vi "save_wav_as_txt.vi"(9 "文件夹名":string, 10 "txt名":string, 11 "wav":dbl[](array[numeric]) caption="一维数据") -> ()   [LabVIEW 2018]
uses:
  <vilib>/Utility/file.llb/Write Delimited Spreadsheet (DBL).vi
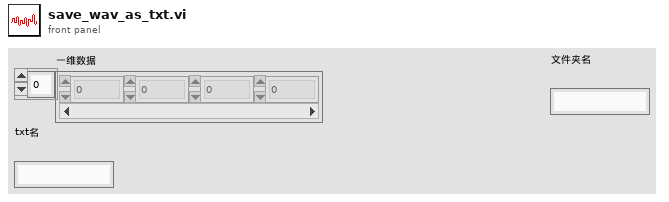
[diagram p1: front panel]
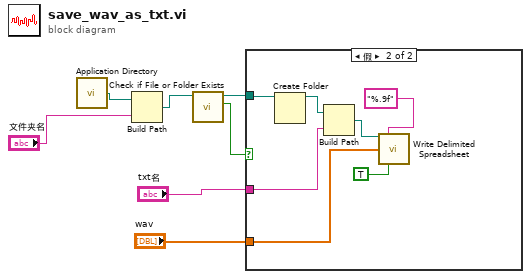
[diagram p0: block diagram]
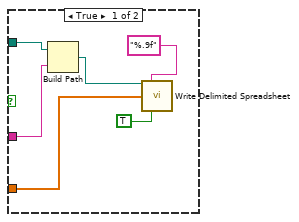
[diagram p2: hidden frame]
diagram:
  n1 = call <vilib>:"Application Directory.vi"() -> ("Application Directory"=w1:path)
  n2 = Build Path(base path=w1, name or relative path="文件夹名") -> (appended path=w6:path)
  n3 = call <vilib>:"Check if File or Folder Exists.vi"("path"=w6) -> ("file or folder exists?"=w5:bool, "dup path"=w3:path)  [unwired: 8 in, 1 out]
  n4 = case shown="假" w5 {
    tunnel: "wav" -> [w11 w18]
    tunnel: w3 -> [w10 w17]
    tunnel: "txt名" -> [w9 w15]
    frame True {
      n5 = Build Path(base path=w10, name or relative path=w9) -> (appended path=w8:path)
      n6 = call-poly <vilib>:"Write Delimited Spreadsheet.vi"("file path (dialog if empty)"=w8, "format (%.3f)"="%.9f", "1D data"=w11, "transpose? (no:F)"=TRUE) -> ()  [unwired: 10 in, 2 out]
    }
    frame False {
      n7 = Create Folder(path (use dialog)=w17) -> (created path=w16:path)  [unwired: 2 in, 2 out]
      n8 = Build Path(base path=w16, name or relative path=w15) -> (appended path=w14:path)
      n9 = call-poly <vilib>:"Write Delimited Spreadsheet.vi"("file path (dialog if empty)"=w14, "format (%.3f)"="%.9f", "1D data"=w18, "transpose? (no:F)"=TRUE) -> ()  [unwired: 10 in, 2 out]
    }
  }
